vi "test-AprilTag-Test1.vi"() -> (3 "All Passed":bool)   [LabVIEW 2019]
uses:
  <vilib>/Rock Robotics/WPI/ThirdParty/JAS_Junk/TrajLib/TypeDef/AprilTagFieldLayout.ctl
  <vilib>/Rock Robotics/WPI/ThirdParty/JAS_Junk/TrajLib/TypeDef/AprilTag.ctl
  <vilib>/Rock Robotics/WPI/ThirdParty/JAS_Junk/TrajLib/TypeDef/POSE3D.ctl
  <vilib>/Rock Robotics/WPI/ThirdParty/JAS_Junk/TrajLib/TypeDef/TRANSLATION3D.ctl
  <vilib>/Rock Robotics/WPI/ThirdParty/JAS_Junk/TrajLib/TypeDef/ROTATION3D.ctl
  <vilib>/Rock Robotics/WPI/ThirdParty/JAS_Junk/TrajLib/TypeDef/QUATERNION.ctl
  <vilib>/Rock Robotics/WPI/ThirdParty/JAS_Junk/TrajLib/Enum/AprilTagFieldLayoutOrignPosition_ENUM.ctl
  <vilib>/Rock Robotics/WPI/ThirdParty/JAS_Junk/TrajLib/Conv_Deg_Radians.vi
  <vilib>/Rock Robotics/WPI/ThirdParty/JAS_Junk/TrajLib/VI/Quaternion_New.vi
  <vilib>/Rock Robotics/WPI/ThirdParty/JAS_Junk/TrajLib/VI/Translation3d_Create.vi
  <vilib>/Rock Robotics/WPI/ThirdParty/JAS_Junk/TrajLib/VI/Pose3d_New_Trans3dRot3d.vi
  <vilib>/Rock Robotics/WPI/ThirdParty/JAS_Junk/TrajLib/VI/AprilTag_GetAll.vi
  <vilib>/Rock Robotics/WPI/ThirdParty/JAS_Junk/TrajLib/Trajectory_Library.lvlib
panel:
  out "AprilTagFieldLayout":T1={"AprilTagMap"={}, "FieldLength"=0.0, "FieldWidth"=0.0, "OriginPosition "=enum."kBlueAllianceWallRightSide,", "OriginPose3d"={"Translation3d"={"X"=0.0, "Y"=0.0, "Z"=0.0}, "Rotation3d"={"Q_quaternion"={"R"=1.0, "V"=[0.0, 0.0, 0.0]}}}} {"OriginPose3d"."Translation3d"."Z" format="%14.3f"; "OriginPose3d"."Translation3d"."Y" format="%14.3f"; "OriginPose3d"."Translation3d"."X" format="%14.3f"}
  out "Test 1 passed":bool
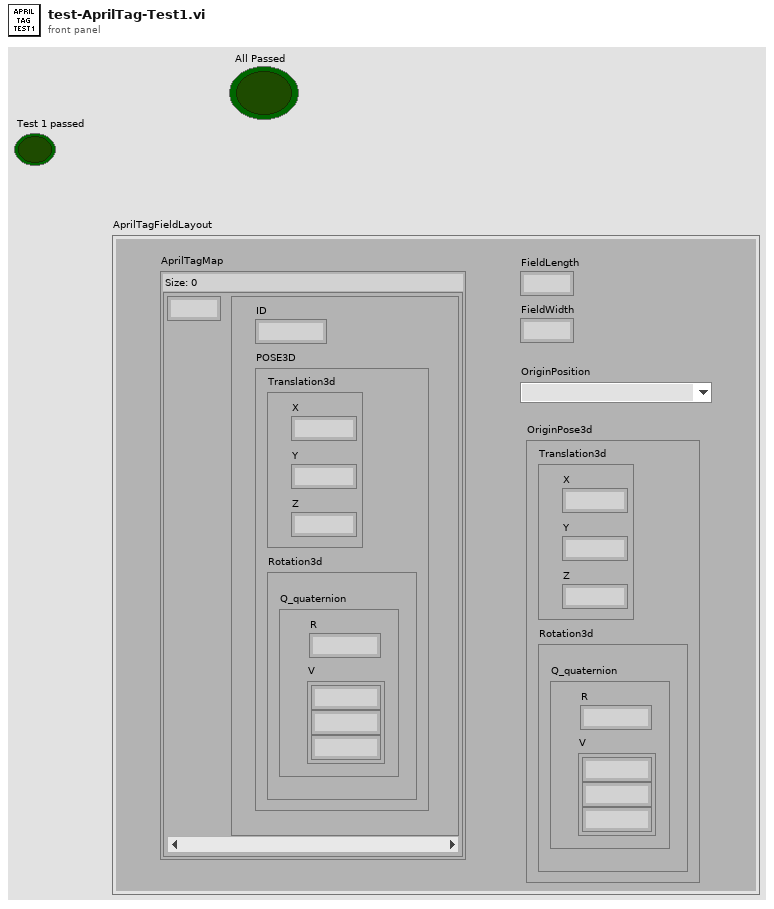
[diagram p1: front panel]
types:
  T1 = typedef "Trajectory_Library.lvlib/AprilTagFieldLayout.ctl" = cluster{"AprilTagMap":map{i32, T2}, "FieldLength":dbl, "FieldWidth":dbl, "OriginPosition ":T7, "OriginPose3d":T3}
  T2 = typedef "Trajectory_Library.lvlib/AprilTag.ctl" = cluster{"ID":i32, "POSE3D":T3}
  T3 = typedef "Trajectory_Library.lvlib/POSE3D.ctl" = cluster{"Translation3d":T4, "Rotation3d":T5}
  T4 = typedef "Trajectory_Library.lvlib/TRANSLATION3D.ctl" = cluster{"X":dbl, "Y":dbl, "Z":dbl}
  T5 = typedef "Trajectory_Library.lvlib/ROTATION3D.ctl" = cluster{"Q_quaternion":T6}
  T6 = typedef "Trajectory_Library.lvlib/QUATERNION.ctl" = cluster{"R":dbl, "V":dbl[]}
  T7 = typedef "Trajectory_Library.lvlib/AprilTagFieldLayoutOrignPosition_ENUM.ctl" = enum16{"kBlueAllianceWallRightSide,", "kRedAllianceWallRightSide,"}
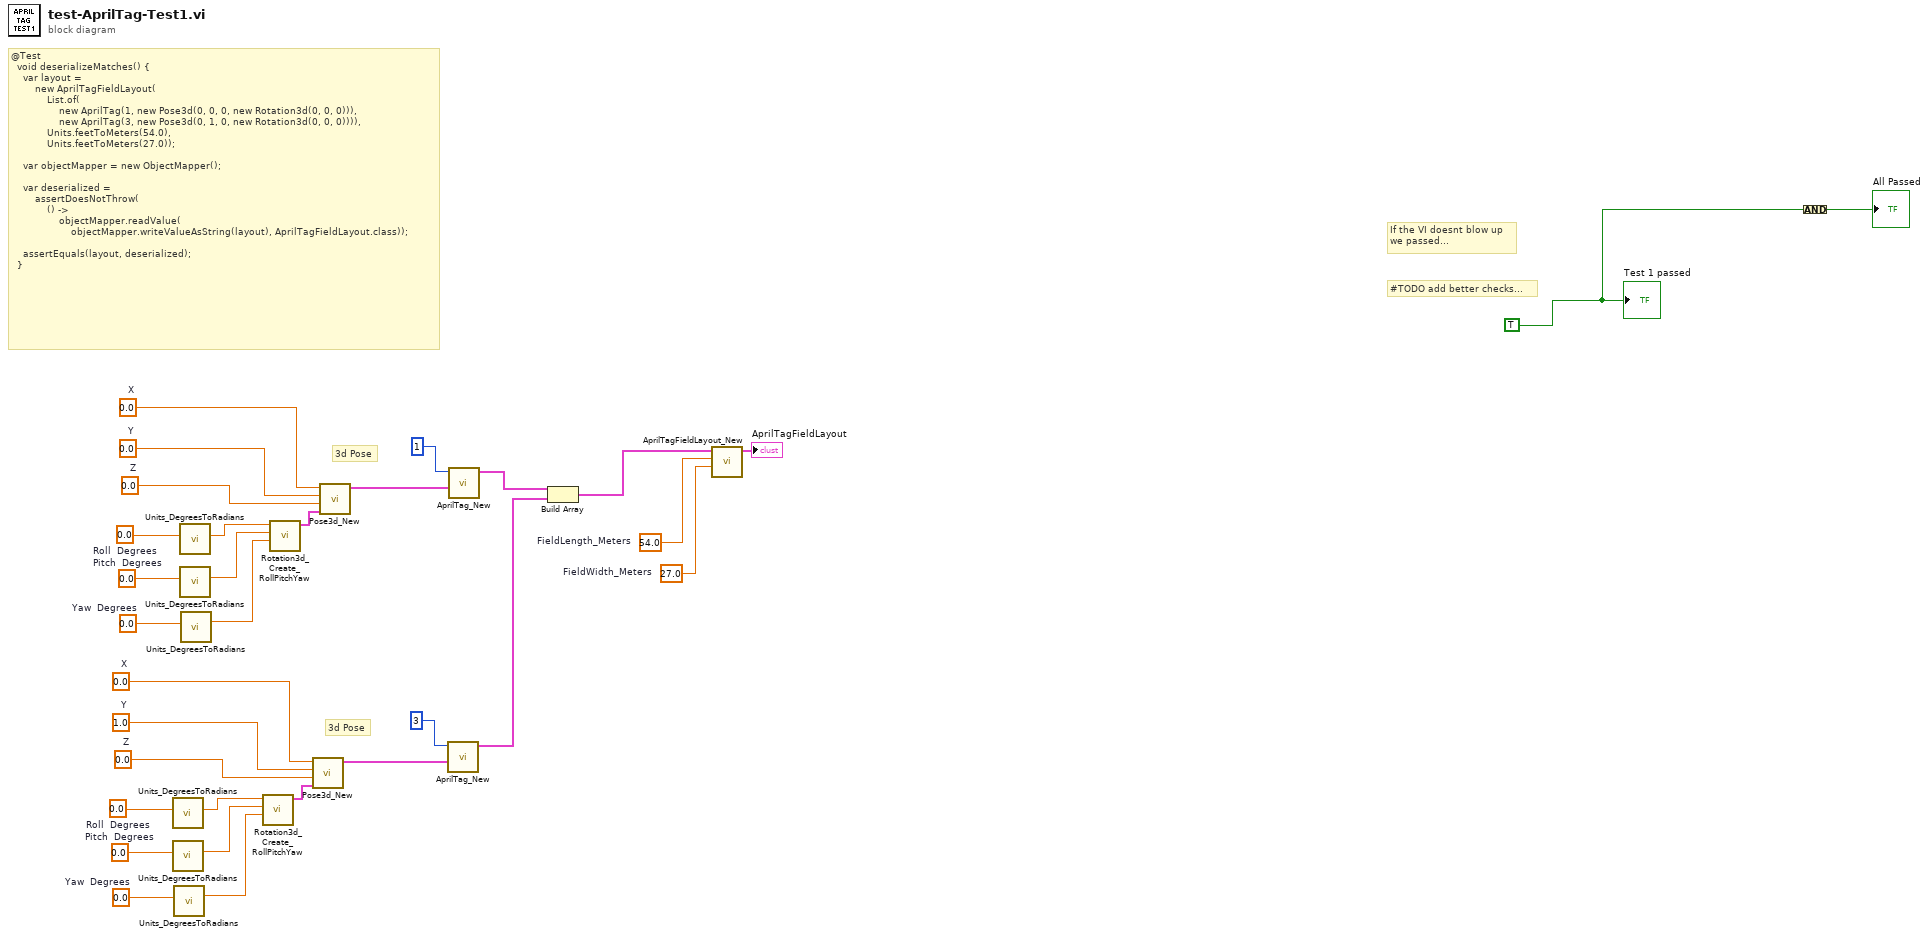
[diagram p0: block diagram]
diagram:
  w1 = TRUE ("Dist To Targ 1")
  w3 = 54.0  # FieldLength_Meters
  w4 = 27.0  # FieldWidth_Meters
  w20 = 0.0  # X
  w19 = 1.0  # Y
  w18 = 0.0  # Z
  w12 = 0.0  # Roll  Degrees
  w13 = 0.0  # Pitch  Degrees
  w14 = 0.0  # Yaw  Degrees
  w30 = 0.0  # X
  w29 = 0.0  # Y
  w28 = 0.0  # Z
  w22 = 0.0  # Roll  Degrees
  w23 = 0.0  # Pitch  Degrees
  w24 = 0.0  # Yaw  Degrees
  # "#TODO add better checks..."
  # "If the VI doesnt blow up\nwe passed..."
  # "3d Pose"
  # "3d Pose"
  # "@Test\n  void deserializeMatches() {\n    var layout =\n        new AprilTagFieldLayout(\n            List.of(\n                new AprilTag(1, new Pose3d(0, 0, 0, new Rotation3d(0, 0, 0))),\n                new AprilTag(3, new Pose3d(0, 1, 0, new Rotation3d(0, 0, 0)))),\n            Units.feetToMeters(54.0),\n            Units.feetToMeters(27.0));\n\n    var objectMapper = new ObjectMapper();\n\n    var deserialized =\n        assertDoesNotThrow(\n            () ->\n                objectMapper.readValue(\n                    objectMapper.writeValueAsString(layout), AprilTagFieldLayout.class));\n\n    assertEquals(layout, deserialized);\n  }"
  n1 = call <vilib>:"Units_DegreesToRadians.vi"("Degrees"=w12) -> ("Radians"=w15:dbl)  [unwired: 10 in]
  n2 = call <vilib>:"Units_DegreesToRadians.vi"("Degrees"=w13) -> ("Radians"=w16:dbl)  [unwired: 10 in]
  n3 = call <vilib>:"Units_DegreesToRadians.vi"("Degrees"=w14) -> ("Radians"=w17:dbl)  [unwired: 10 in]
  n4 = call <vilib>:"Units_DegreesToRadians.vi"("Degrees"=w22) -> ("Radians"=w25:dbl)  [unwired: 10 in]
  n5 = call <vilib>:"Units_DegreesToRadians.vi"("Degrees"=w23) -> ("Radians"=w26:dbl)  [unwired: 10 in]
  n6 = call <vilib>:"Units_DegreesToRadians.vi"("Degrees"=w24) -> ("Radians"=w27:dbl)  [unwired: 10 in]
  n7 = call <vilib>:"Rotation3d_Create_RollPitchYaw.vi"("Yaw"=w17, "Pitch"=w16, "Roll"=w15) -> ("Rotation3d"=w21:T5)  [unwired: 8 in]
  n8 = call <vilib>:"Rotation3d_Create_RollPitchYaw.vi"("Yaw"=w27, "Pitch"=w26, "Roll"=w25) -> ("Rotation3d"=w31:T5)  [unwired: 8 in]
  n9 = call <vilib>:"Pose3d_New.vi"("Rotation3d"=w21, "z"=w18, "Y"=w19, "X"=w20) -> ("out Pose3d"=w8:T3)  [unwired: 7 in]
  n10 = call <vilib>:"Pose3d_New.vi"("Rotation3d"=w31, "z"=w28, "Y"=w29, "X"=w30) -> ("out Pose3d"=w10:T3)  [unwired: 7 in]
  n11 = call <vilib>:"AprilTag_New.vi"("POSE3D"=w8, "ID"=3) -> ("AprilTag"=w6:T2)  [unwired: 9 in]
  n12 = call <vilib>:"AprilTag_New.vi"("POSE3D"=w10, "ID"=1) -> ("AprilTag"=w7:T2)  [unwired: 9 in]
  n13 = Build Array(w7, w6) -> (w5:T2[])
  n14 = call <vilib>:"AprilTagFieldLayout_New.vi"("FieldWidth_Meters"=w4, "FieldLength_Meters"=w3, "AprilTags"=w5) -> ("AprilTagFieldLayout"=→"AprilTagFieldLayout":T1)  [unwired: 8 in]
  n15 = Compound Arithmetic op=AND(w1) -> (→"All Passed":bool)
  "Test 1 passed" <- w1
